vi "Run Project Unit Tests (Caraya).vi"(6 "Variant in":variant, 7 "Shift Pressed?":bool, 8 "error in (no error)":errorcluster, 10 "QD Combo Box Ref":refnum<vi>, 11 "QD Launch VI Ref":refnum<vi>) -> (0 "error out":errorcluster, 4 "Variant out":variant)   [LabVIEW 2013]
doc: "This QD shortcut will discover all the Caraya Unit Tests in a project and run them in interactive mode.\n(Optional best match for virtual folder from the text in the combo box)\n\nDefault Shortcut - [U]"
uses:
  classes/Test Runner/Test Runner.lvclass/Test Runner.ctl
  classes/Test Runner.Project/Test Runner.Project.lvclass
  classes/Test Runner/Test Runner.lvclass
  classes/Test Runner.Folder/Test Runner.Folder.lvclass
panel:
  out "Test VIs":path[](array[path])
  in  "Undo Name":string="Run Project Unit Tests"
  # "Do not change the connector pane of this VI.\n\nSee the block diagram for directions on how to use this template."
  # "Specify the name of the Undo transaction"
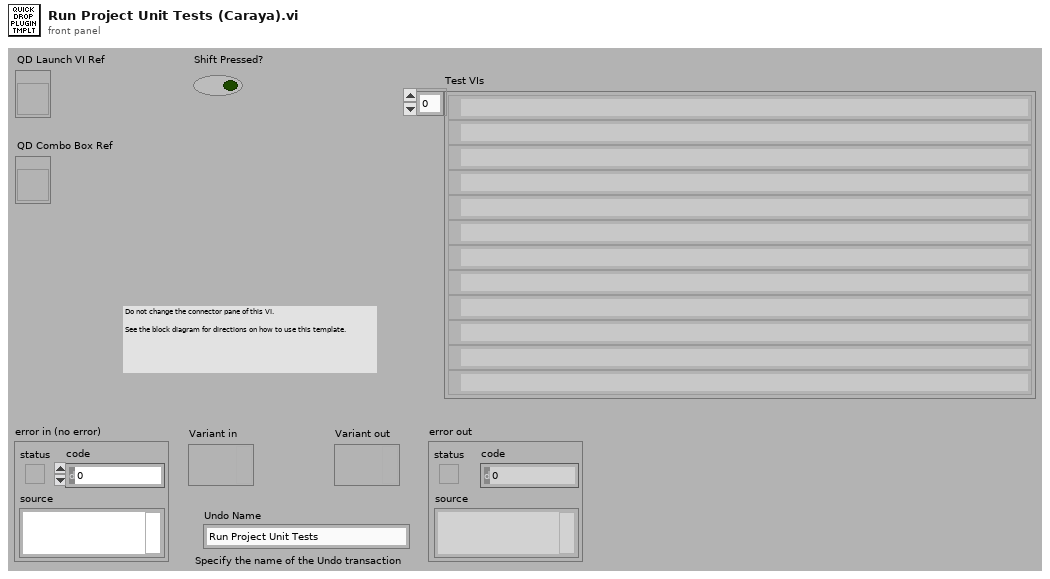
[diagram p1: front panel]
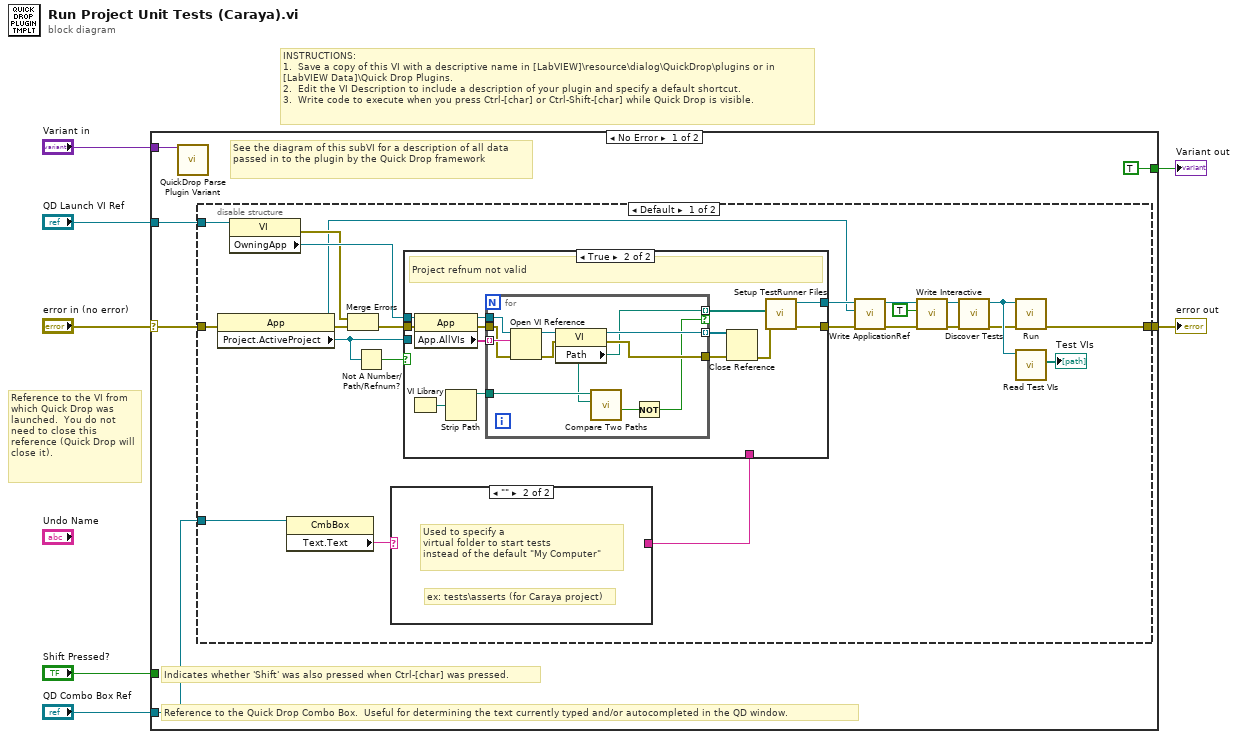
[diagram p0: block diagram]
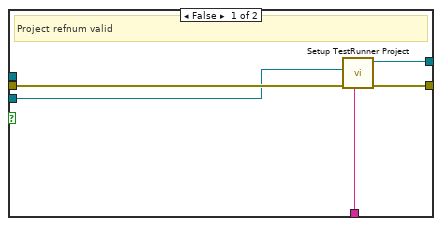
[diagram p2: hidden frame]
diagram:
  # "Reference to the VI from which Quick Drop was launched.  You do not need to close this reference (Quick Drop will close it)."
  # "INSTRUCTIONS:\n1.  Save a copy of this VI with a descriptive name in [LabVIEW]\\resource\\dialog\\QuickDrop\\plugins or in [LabVIEW Data]\\Quick Drop Plugins.\n2.  Edit the VI Description to include a description of your plugin and specify a default shortcut. \n3.  Write code to execute when you press Ctrl-[char] or Ctrl-Shift-[char] while Quick Drop is visible."
  n1 = case shown="No Error" "error in (no error)" {
    selector: "error in (no error)" -> [w11 w67]
    tunnel: [w9 w67] -> w6
    tunnel: "QD Launch VI Ref" -> [w8 _]
    tunnel: "Shift Pressed?" -> [_ _]
    tunnel: "QD Combo Box Ref" -> [w10 _]
    tunnel: "Variant in" -> [w13 _]
    tunnel: [TRUE _] -> w1
    frame No Error {
      # "See the diagram of this subVI for a description of all data passed in to the plugin by the Quick Drop framework"
      # "Reference to the Quick Drop Combo Box.  Useful for determining the text currently typed and/or autocompleted in the QD window."
      # "Indicates whether 'Shift' was also pressed when Ctrl-[char] was pressed."
      n2 = call <vilib>:"QuickDrop Parse Plugin Variant.vi"("QDKS Variant in"=w13) -> ()  [unwired: 12 in, 3 out]
      n3 = disable-structure shown="Default" {
        disable-tunnel: w11 -> [w35 w66]
        disable-tunnel: w10 -> [w34 _]
        disable-tunnel: [w26 w66] -> w9
        disable-tunnel: w8 -> [w19 _]
        frame condition #0 (active) {
          n4 = property on="Property Node" class="App"(error in=w35) -> (reference out=w14:refnum<vi>, error out=w16:errorcluster, "Project.ActiveProject"=w21:refnum<vi>)  [unwired: 1 in]
          n5 = property on="Property Node" class="VI"(reference=w19) -> (error out=w17:errorcluster, "OwningApp"=w18:refnum<vi>)  [unwired: 1 in, 1 out]
          n6 = property on="Property Node" class="CmbBox"(reference=w34) -> ("Text.Text"=w33:string)  [unwired: 1 in, 2 out]
          n7 = Merge Errors(w17, w16) -> (w15:errorcluster)
          n8 = Not A Number/Path/Refnum?(number/path/refnum=w21) -> (NaN/Path/Refnum?=w20:bool)
          n9 = case shown="\"\"" w33 {
            selector: w33 -> [w65 _]
            tunnel: [w65 _] -> w29
            frame Default {
            }
            frame "" {
              # "ex: tests\\asserts (for Caraya project)"
              # "Used to specify a\nvirtual folder to start tests\ninstead of the default \"My Computer\""
            }
          }
          n10 = case shown="True" w20 {
            tunnel: w29 -> [w40 _]
            tunnel: [w39 w52] -> w25
            tunnel: [w38 w51] -> w23
            tunnel: w15 -> [w37 w53]
            tunnel: w21 -> [w36 _]
            tunnel: w18 -> [_ w43]
            frame False {
              # "Project refnum valid"
              n11 = call "Setup TestRunner Project.vi"("Virtual Folder (empty: \"My Computer\")"=w40, "error in (no error)"=w37, "Project Refnum"=w36) -> ("error out"=w38:errorcluster, "Test Runner.Project out"=w39:refnum<class "Test Runner.Project.lvclass">)  [unwired: 7 in]
            }
            frame True {
              # "Project refnum not valid"
              n12 = VI Library() -> (path=w46:path)
              n13 = property class="App"(reference=w43, error in=w53) -> (reference out=w42:refnum<vi>, error out=w41:errorcluster, "App.AllVIs"=w50:string[])
              n14 = Strip Path(path=w46) -> (stripped path=w45:path)  [unwired: 1 out]
              n15 = for {
                tunnel: w50 -> [w64] mode=indexing
                tunnel: [w62] -> w49 mode=indexing
                tunnel: [w58] -> w44 mode=indexing if=w56
                tunnel: [w60] -> w48
                tunnel: w45 -> [w59]
                tunnel: w42 -> [w55]
                tunnel: w41 -> [w54]
                n16 = Open VI Reference(application reference (local)=w55, vi path=w64, error in (no error)=w54) -> (vi reference=w63:refnum<vi>, error out=w61:errorcluster)  [unwired: 3 in]
                n17 = property class="VI"(reference=w63, error in=w61) -> (reference out=w62:refnum<vi>, error out=w60:errorcluster, "Path"=w58:path)
                n18 = call <vilib>:"Compare Two Paths.vi"("Path 2"=w58, "Path 1"=w59) -> ("Path 2 Relative to Path 1?"=w57:bool)  [unwired: 6 in, 3 out]
                n19 = Not(x=w57) -> (.not. x?=w56:bool)
              }
              n20 = Close Reference(reference=w49, error in (no error)=w48) -> (error out=w47:errorcluster)
              n21 = call "Setup TestRunner Files.vi"("error in (no error)"=w47, "Paths"=w44) -> ("error out"=w51:errorcluster, "Test Runner.Folder out"=w52:refnum<class "Test Runner.Folder.lvclass">)  [unwired: 8 in]
            }
          }
          n22 = call "Write ApplicationRef.vi"("error in (no error)"=w23, "Application"=w14, "Test Runner in"=w25) -> ("error out"=w22:errorcluster, "Test Runner out"=w24:refnum<class "Test Runner.lvclass">)  [unwired: 7 in]
          n23 = call "Write Interactive.vi"("Interactive"=TRUE, "Test Runner in"=w24) -> ("Test Runner out"=w31:refnum<class "Test Runner.lvclass">)  [unwired: 9 in]
          n24 = call "Discover Tests.vi"("error in (no error)"=w22, "Test Runner in"=w31) -> ("error out"=w27:errorcluster, "Test Runner out"=w28:refnum<class "Test Runner.lvclass">)  [unwired: 8 in]
          n25 = call "Run.vi"("error in (no error)"=w27, "Test Runner in"=w28) -> ("error out"=w26:errorcluster)  [unwired: 8 in, 1 out]
          n26 = call "Read Test VIs.vi"("Test Runner in"=w28) -> ("Test VIs"=→"Test VIs":path[])  [unwired: 8 in, 2 out]
        }
        frame condition #1 {
        }
      }
    }
    frame Error {
    }
  }
  "error out" <- w6
  "Variant out" <- w1
